vi "SVT DC Motor.vi"(0 "nominal speed [RPM]":dbl=1800.0, 1 "desired units":u16(ring) items=["Hz", "Order"], 5 "line frequency [Hz]":dbl=60.0, 11 "error in (no error)":errorcluster) -> (4 "frequency of silicon-controlled rectifier (full-wave)":dbl=360.0, 6 "frequency of silicon-controlled rectifier (half-wave)":dbl=180.0, 15 "error out":errorcluster)   [LabVIEW 2017, in "SoundVib_MachineCharacteristic.lvlib"]
doc: "Calculates characteristic frequencies or orders of motors. You must manually select the polymorphic instance you want to use."
uses:
  <vilib>/addons/Sound and Vibration/svt_Machine Characteristic/SoundVib_MachineCharacteristic.lvlib
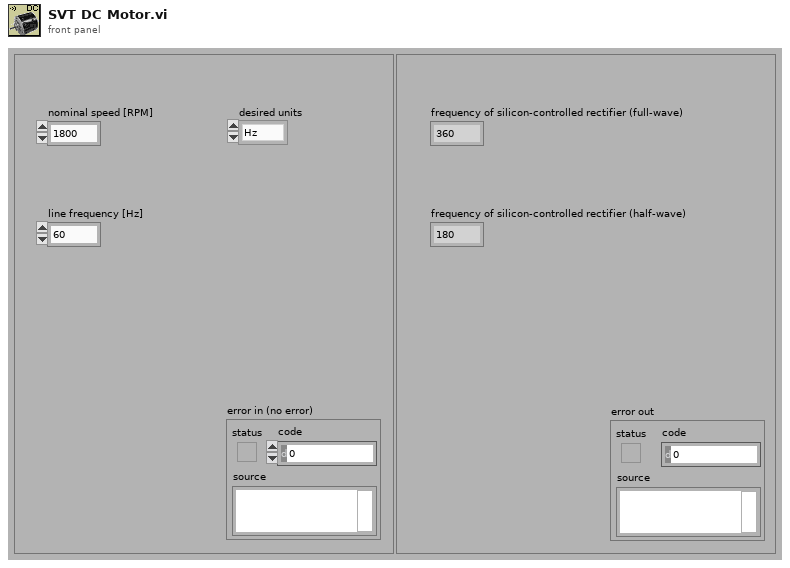
[diagram p1: front panel]
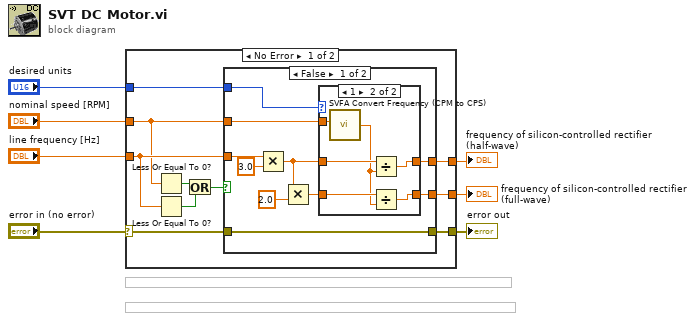
[diagram p0: block diagram]
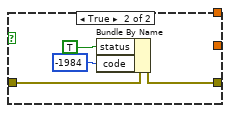
[diagram p3: hidden frame]
diagram:
  n1 = case shown="No Error" "error in (no error)" {
    selector: "error in (no error)" -> [w14 w40]
    tunnel: [w13 w40] -> w6
    tunnel: "line frequency [Hz]" -> [w11 _]
    tunnel: "nominal speed [RPM]" -> [w8 _]
    tunnel: "desired units" -> [w12 _]
    tunnel: [w10 _] -> w2
    tunnel: [w9 _] -> w1
    frame No Error {
      n2 = Less Or Equal To 0?(x=w8) -> (x <= 0?=w17:bool)
      n3 = Less Or Equal To 0?(x=w11) -> (x <= 0?=w16:bool)
      n4 = Or(x=w17, y=w16) -> (x .or. y?=w15:bool)
      n5 = case shown="False" w15 {
        tunnel: w14 -> [w27 w39]
        tunnel: [w27 w38] -> w13
        tunnel: w12 -> [w23 _]
        tunnel: w11 -> [w26 _]
        tunnel: [w20 _] -> w10
        tunnel: [w19 _] -> w9
        tunnel: w8 -> [w18 _]
        frame False {
          n6 = Multiply(x=w26, y=3.0) -> (x*y=w22:dbl)
          n7 = Multiply(x=w22, y=2.0) -> (x*y=w21:dbl)
          n8 = case shown="1" w23 {
            tunnel: [w29 w33] -> w20
            tunnel: w22 -> [w29 w35]
            tunnel: [w28 w32] -> w19
            tunnel: w21 -> [w28 w34]
            tunnel: w18 -> [_ w31]
            frame 0, Default {
            }
            frame 1 {
              n9 = call <vilib>:"SVFA Convert Frequency (CPM to CPS).vi"("nominal speed [RPM]"=w31) -> ("frequency [Hz]"=w30:dbl)  [unwired: 5 in]
              n10 = Divide(x=w35, y=w30) -> (x/y=w33:dbl)
              n11 = Divide(x=w34, y=w30) -> (x/y=w32:dbl)
            }
          }
        }
        frame True {
          n12 = Bundle By Name(cluster=w39, "status"=TRUE, "code"=-1984) -> (w38:errorcluster)
        }
      }
    }
    frame Error {
    }
  }
  "frequency of silicon-controlled rectifier (full-wave)" <- w1
  "error out" <- w6
  "frequency of silicon-controlled rectifier (half-wave)" <- w2
